vi "Get Via App.vi"(8 "error in (no error)":errorcluster, 11 "GWebAppArrayPanel in":refnum<class "GWebAppArrayPanel.lvclass">) -> (0 "error out":errorcluster, 2 "App":refnum<class "ViaApp.lvclass">, 3 "GWebAppArrayPanel out":refnum<class "GWebAppArrayPanel.lvclass">)   [LabVIEW 2020, in "PicoG-App.lvlib" / "GWebAppArrayPanel.lvclass"]
uses:
  GWebAppArrayPanel.lvclass
  ViaApp/ViaApp.lvclass
  GWebAppArrayPanel.lvclass/GWebAppArrayPanel.ctl
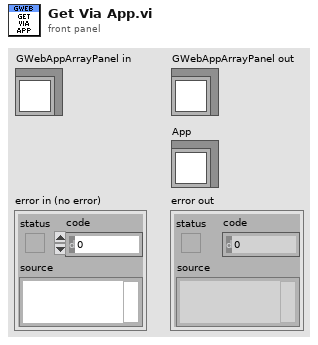
[diagram p1: front panel]
types:
  T1 = typedef "PicoG-App.lvlib/GWebAppArrayPanel.lvclass/Ref Data.ctl" = cluster{"App":refnum<class "ViaApp.lvclass">}
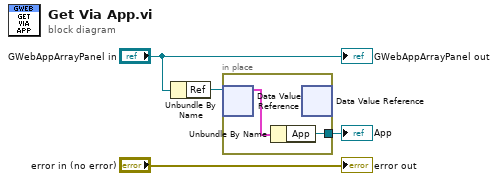
[diagram p0: block diagram]
diagram:
  n1 = Unbundle By Name("GWebAppArrayPanel in") -> ("Ref"=w3:refnum<data-value>)
  n2 = in-place {
    in-place-border: [w5] -> w1
    n3 = in-place-dvr #1(w3) -> (w6:T1)  [unwired: 1 out]
    n4 = Unbundle By Name(w6) -> ("App"=w5:refnum<class "ViaApp.lvclass">)
    n5 = in-place-dvr #1() -> ()  [unwired: 1 in, 2 out]
  }
  "App" <- w1
  "error out" <- "error in (no error)"
  "GWebAppArrayPanel out" <- "GWebAppArrayPanel in"
